vi "ddsDirectionArrayConvert.vi"(7 "Pre 3.0 AOM driver version?":bool, 10 "Register":dbl=9.0 min=0.0 max=15.0 step=1.0 format="%#.1f", 11 "Direction (0 = down; 1 = up)":dbl[](array[numeric])=[0.0] min=0.0 max=1.0 step=1.0 format="%#.0g") -> (3 "Characters for FPGA":string="L90\r\n")   [LabVIEW 2013, in "DDS9954_v2013.lvlib"]
uses:
  DDS9954_v2013.lvlib
  dataToAscii_8bit.vi
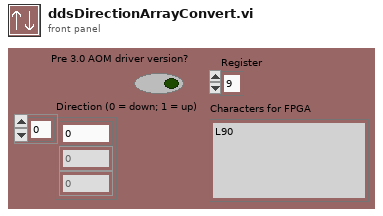
[diagram p1: front panel]
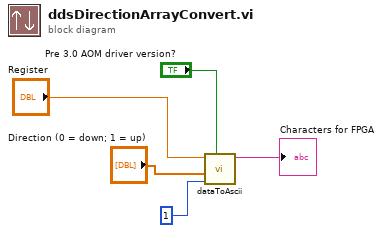
[diagram p0: block diagram]
diagram:
  n1 = call-poly "dataToAscii.vi"("Pre 3.0 AOM driver version?"="Pre 3.0 AOM driver version?", "HEX min width (pre 3.0)"=u8 1, "Input Data"="Direction (0 = down; 1 = up)", "Register"="Register") -> ("Characters to FPGA"=→"Characters for FPGA":string)  [unwired: 7 in]
